vi "Split and Merge Test.vi"() -> ()   [LabVIEW 2017]
panel:
  in  "stop":bool
  out "XY Graph 2":cluster{dbl[], dbl[]}[](graph)
  in  "Threshold":dbl
  in  "Threshold":dbl
  out "XY Graph":cluster{dbl[], dbl[]}(graph)
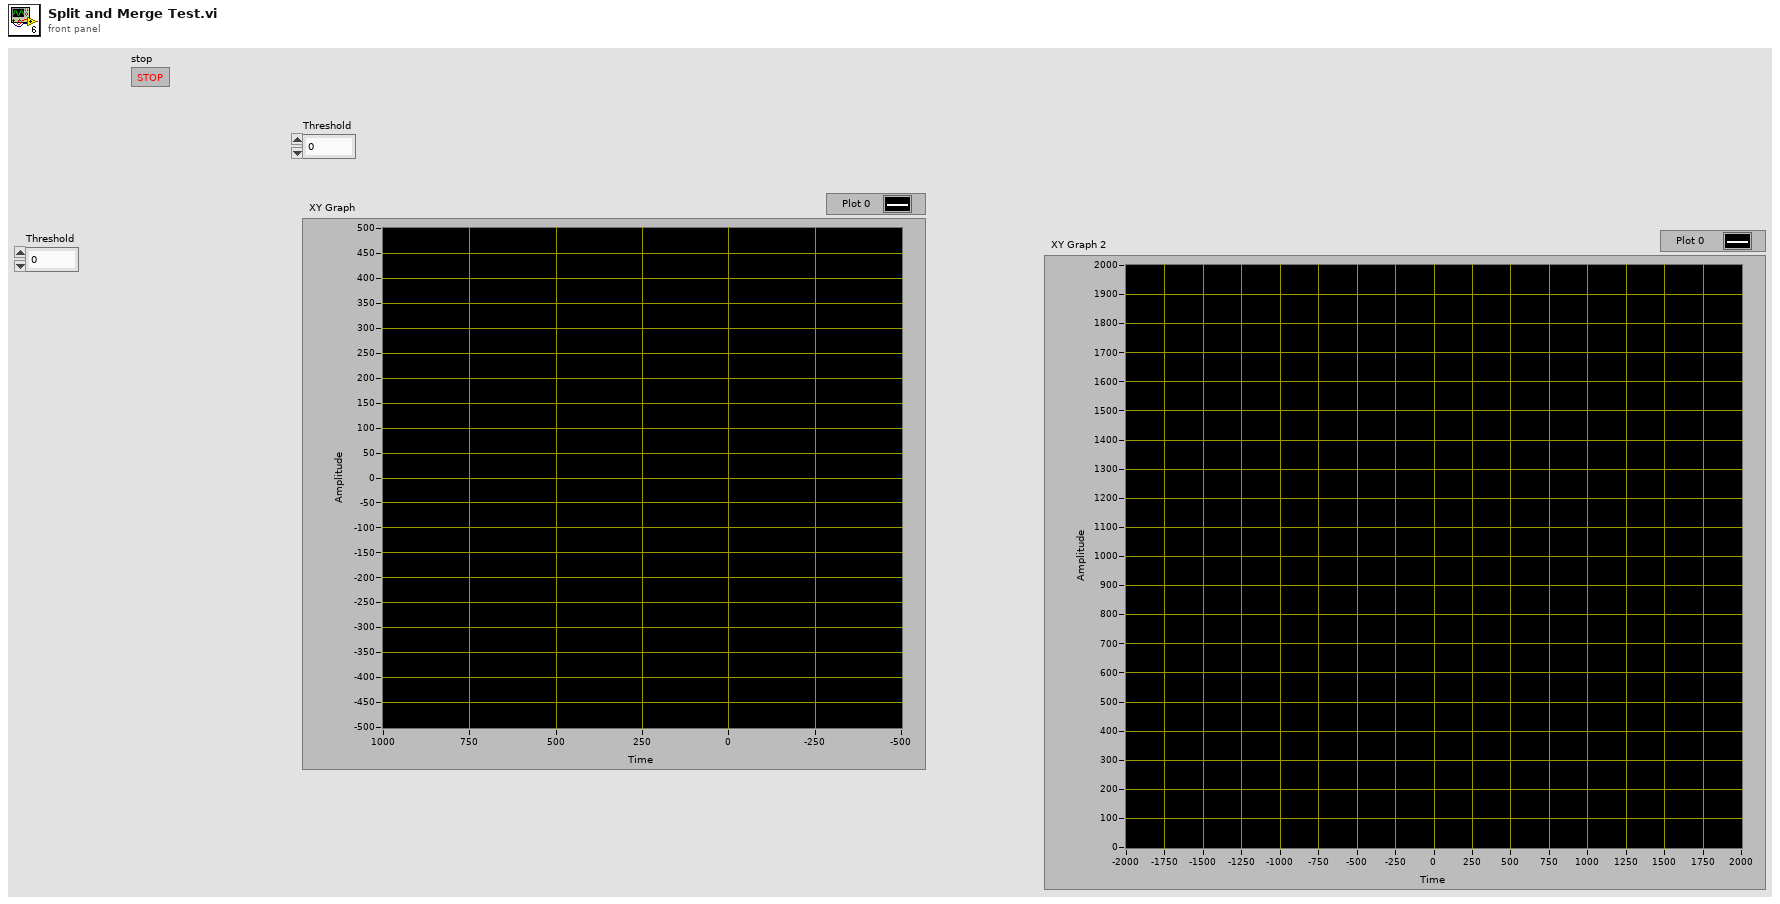
[diagram p1: front panel]
types:
  T1 = typedef "LidarPoint.ctl" = cluster{"X":dbl, "Y":dbl}
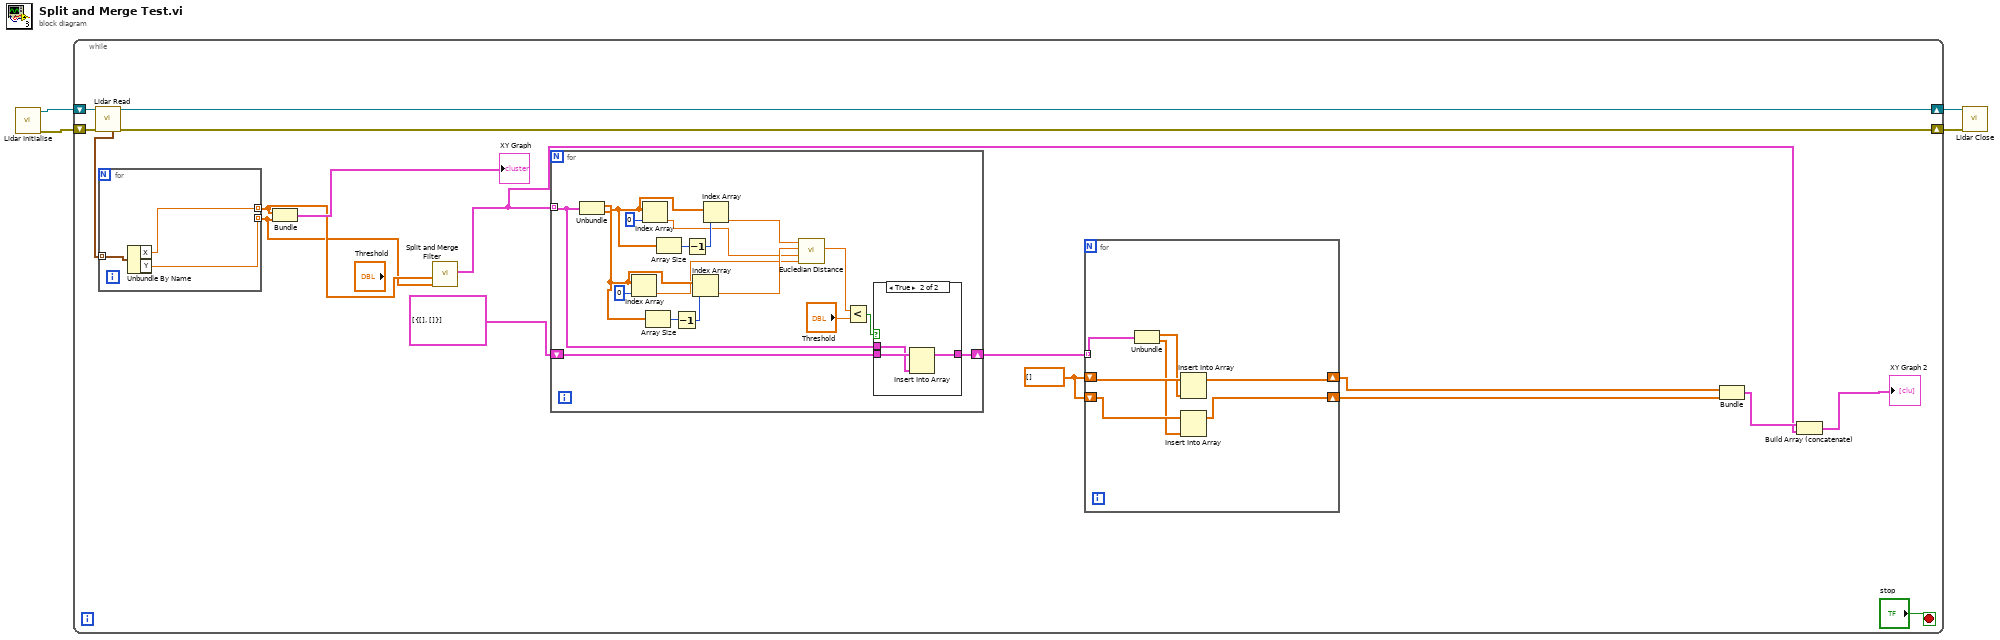
[diagram p0: block diagram]
diagram:
  n1 = call "Lidar Initialise.vi"() -> ("error out"=w2:errorcluster, "VISA resource name out"=w4:refnum<visa-resource-name>)  [unwired: 10 in]
  n2 = while {
    shift-right: [w20] -> w3
    shift-left: w4 -> [w21]
    shift-right: [w18] -> w1
    shift-left: w2 -> [w19]
    stop <- "stop" stop-if-true
    w12 = dbl[] []
    n3 = call "Lidar Read.vi"("error in (no error)"=w19, "VISA resource name"=w21) -> ("error out"=w18:errorcluster, "VISA resource name out"=w20:refnum<visa-resource-name>, "square"=w8:T1[])  [unwired: 2 in, 4 out]
    n4 = for {
      tunnel: w8 -> [w53] mode=indexing
      tunnel: [w52] -> w16 mode=indexing
      tunnel: [w51] -> w15 mode=indexing
      n5 = Unbundle By Name(w53) -> ("X"=w52:dbl, "Y"=w51:dbl)
    }
    n6 = Bundle(w16, w15) -> (→"XY Graph":cluster{dbl[], dbl[]})  [unwired: 1 in]
    n7 = call "Split and Merge Filter.vi"("Y"=w15, "X"=w16) -> ("Array"=w5:cluster{dbl[], dbl[]}[])  [unwired: 9 in]
    n8 = for {
      tunnel: w5 -> [w29] mode=indexing
      shift-right: [w30] -> w13
      shift-left: cluster{dbl[], dbl[]}[] [{[], []}] ("Array 2") -> [w31]
      n9 = Unbundle(w29) -> (w45:dbl[], w39:dbl[])
      n10 = Index Array(array=w39, index=0) -> (element=w35:dbl)
      n11 = Index Array(array=w45, index=0) -> (element=w36:dbl)
      n12 = Array Size(array=w39) -> (size(s)=w41:i32)
      n13 = Array Size(array=w45) -> (size(s)=w44:i32)
      n14 = Decrement(x=w41) -> (x-1=w42:i32)
      n15 = Decrement(x=w44) -> (x-1=w43:i32)
      n16 = Index Array(array=w39, index=w42) -> (element=w37:dbl)
      n17 = Index Array(array=w45, index=w43) -> (element=w38:dbl)
      n18 = call "Eucledian Distance.vi"("Y2"=w35, "X2"=w36, "Y"=w37, "X"=w38) -> ("Distance"=w34:dbl)  [unwired: 7 in]
      n19 = Less?(x=w34, y="Threshold") -> (x < y?=w33:bool)
      n20 = case shown="True" w33 {
        tunnel: w31 -> [w47 w50]
        tunnel: [w47 w49] -> w30
        tunnel: w29 -> [_ w48]
        frame False {
        }
        frame True {
          n21 = Insert Into Array(array=w50, new element=w48) -> (w49:cluster{dbl[], dbl[]}[])  [unwired: 1 in]
        }
      }
    }
    n22 = for {
      tunnel: w13 -> [w28] mode=indexing
      shift-right: [w23] -> w10
      shift-left: w12 -> [w27]
      shift-right: [w22] -> w9
      shift-left: w12 -> [w26]
      n23 = Unbundle(w28) -> (w24:dbl[], w25:dbl[])
      n24 = Insert Into Array(array=w27, new element=w24) -> (w23:dbl[])  [unwired: 1 in]
      n25 = Insert Into Array(array=w26, new element=w25) -> (w22:dbl[])  [unwired: 1 in]
    }
    n26 = Bundle(w10, w9) -> (w7:cluster{dbl[], dbl[]})  [unwired: 1 in]
    n27 = Build Array (concatenate)(w7, w5) -> (→"XY Graph 2":cluster{dbl[], dbl[]}[])
  }
  n28 = call "Lidar Close.vi"("error in (no error)"=w1, "VISA resource name"=w3) -> ()  [unwired: 9 in, 1 out]
